vi "Generate Trace for Stopped Actor.vi"(10 "Actor Enqueuer":refnum<class "Message Enqueuer.lvclass">) -> ()   [LabVIEW 2020, in "Actor Framework.lvlib"]
doc: "Generates a DETT User Generated Trace for an actor stopping, whether in response to the Stop Msg or an error or its normal termination."
uses:
  vi.lib/ActorFramework/Actor Framework.lvlib
  vi.lib/ActorFramework/Message Enqueuer/Message Enqueuer.lvclass
  vi.lib/ActorFramework/tracing/Support/Registration Mode.ctl
  vi.lib/ActorFramework/tracing/Support/Localized Strings.vi
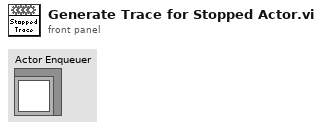
[diagram p1: front panel]
types:
  T1 = typedef "Actor Framework.lvlib/Registration Mode.ctl" = enum16{"Register Actor", "Get ID", "Get Enqueuer", "Deregister Actor", "Get Update Event", "Get All Actors", "Set Actor Core Name"}
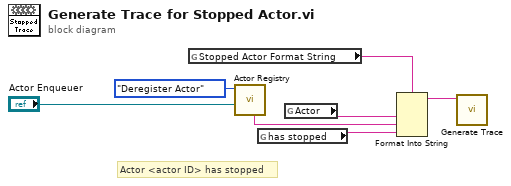
[diagram p0: block diagram]
diagram:
  # "Actor <actor ID> has stopped"
  n1 = global read "Localized Strings.vi" "Stopped Actor Format String"() -> (w2:string)
  n2 = call "Actor Registry.vi"("Actor Enqueuer"="Actor Enqueuer", "Action"=Registration_Mode."Deregister Actor") -> ("Actor Alias out"=w5:string)  [unwired: 5 in, 4 out]
  n3 = global read "Localized Strings.vi" "has stopped"() -> (w3:string)
  n4 = global read "Localized Strings.vi" "Actor"() -> (w4:string)
  n5 = Format Into String(format string=w2, w4, w5, w3) -> (resulting string=w1:string)  [unwired: 2 in, 1 out]
  n6 = call "Generate Trace.vi"("String"=w1) -> ()  [unwired: 11 in]
